vi "Helper Loop Status Updated.vi"(8 "error in":errorcluster, 10 "Helper Loop Status":T1=enum."Asleep", 11 "Module ID":i32=-1) -> (0 "error out":errorcluster)   [LabVIEW 2020, in "Monochromator.lvlib"]
doc: "Helper Loop Status Updated\n_____\nCreated using DQMH Event Scripter 6.1.0.128.\n____\nPantherLAB Templates 1.0.0.1\nCopyright (c) 2022, PantherLAB\n____\nPantherLAB Templates 1.0.0.5\nCopyright (c) 2022, PantherLAB"
uses:
  Monochromator.lvlib
  Helper Loop Status--enum.ctl
  Helper Loop Status Updated Argument--cluster.ctl
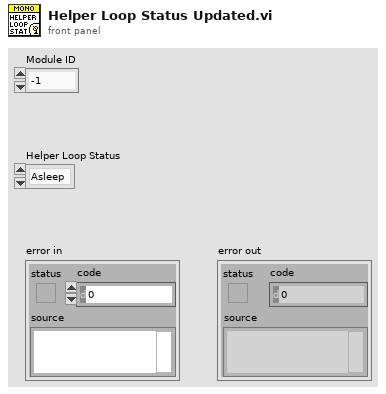
[diagram p1: front panel]
types:
  T1 = typedef "Monochromator.lvlib/Helper Loop Status--enum.ctl" = enum16{"Awake", "Asleep"}
  T2 = typedef "Monochromator.lvlib/Helper Loop Status Updated Argument--cluster.ctl" = cluster{"Module ID":i32, "Helper Loop Status":T1}
  T3 = typedef "Monochromator.lvlib/Broadcast Events--cluster.ctl" = cluster{"Module Did Init":refnum<user-event>, "Status Updated":refnum<user-event>, "Error Reported":refnum<user-event>, "Module Did Stop":refnum<user-event>, "Update Module Execution Status":refnum<user-event>, "Helper Loop Status Updated":refnum<user-event>}
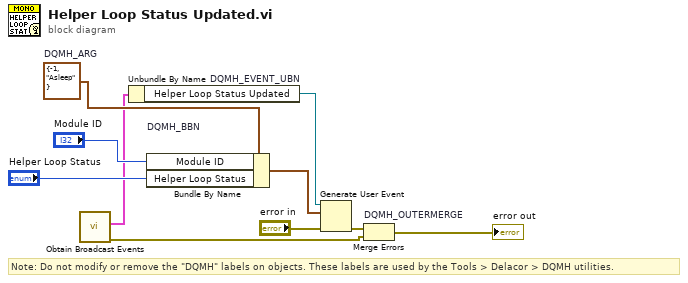
[diagram p0: block diagram]
diagram:
  w5 = T2 {"Module ID"=-1, "Helper Loop Status"=enum."Asleep"}  # DQMH_ARG
  # "Note: Do not modify or remove the \"DQMH\" labels on objects. These labels are used by the Tools > Delacor > DQMH utilities."
  n1 = call "Obtain Broadcast Events.vi"() -> ("error out"=w2:errorcluster, "Monochromator Broadcast Events"=w1:T3)  [unwired: 10 in]
  n2 = Unbundle By Name "DQMH_EVENT_UBN"(w1) -> ("Helper Loop Status Updated"=w7:refnum<user-event>)
  n3 = Bundle By Name "DQMH_BBN"(cluster=w5, "Module ID"="Module ID", "Helper Loop Status"="Helper Loop Status") -> (w8:T2)
  n4 = Generate User Event(user event=w7, event data cluster=w8, error in="error in") -> (error out=w6:errorcluster)  [unwired: 1 in, 1 out]
  n5 = Merge Errors "DQMH_OUTERMERGE"(w6, w2) -> (→"error out":errorcluster)
